vi "ATF-Sequence file decoder.vi"(8 "error in (no error)":errorcluster, 11 "file path (dialog if empty)":path) -> (0 "error out":errorcluster, 3 "Seq in":T1(array[cluster]))   [LabVIEW 2022 SP3]
uses:
  <vilib>/Utility/file.llb/Read Delimited Spreadsheet (string).vi
panel:
  in  "output cluster":T2
  out "all rows":string[][](array[string])
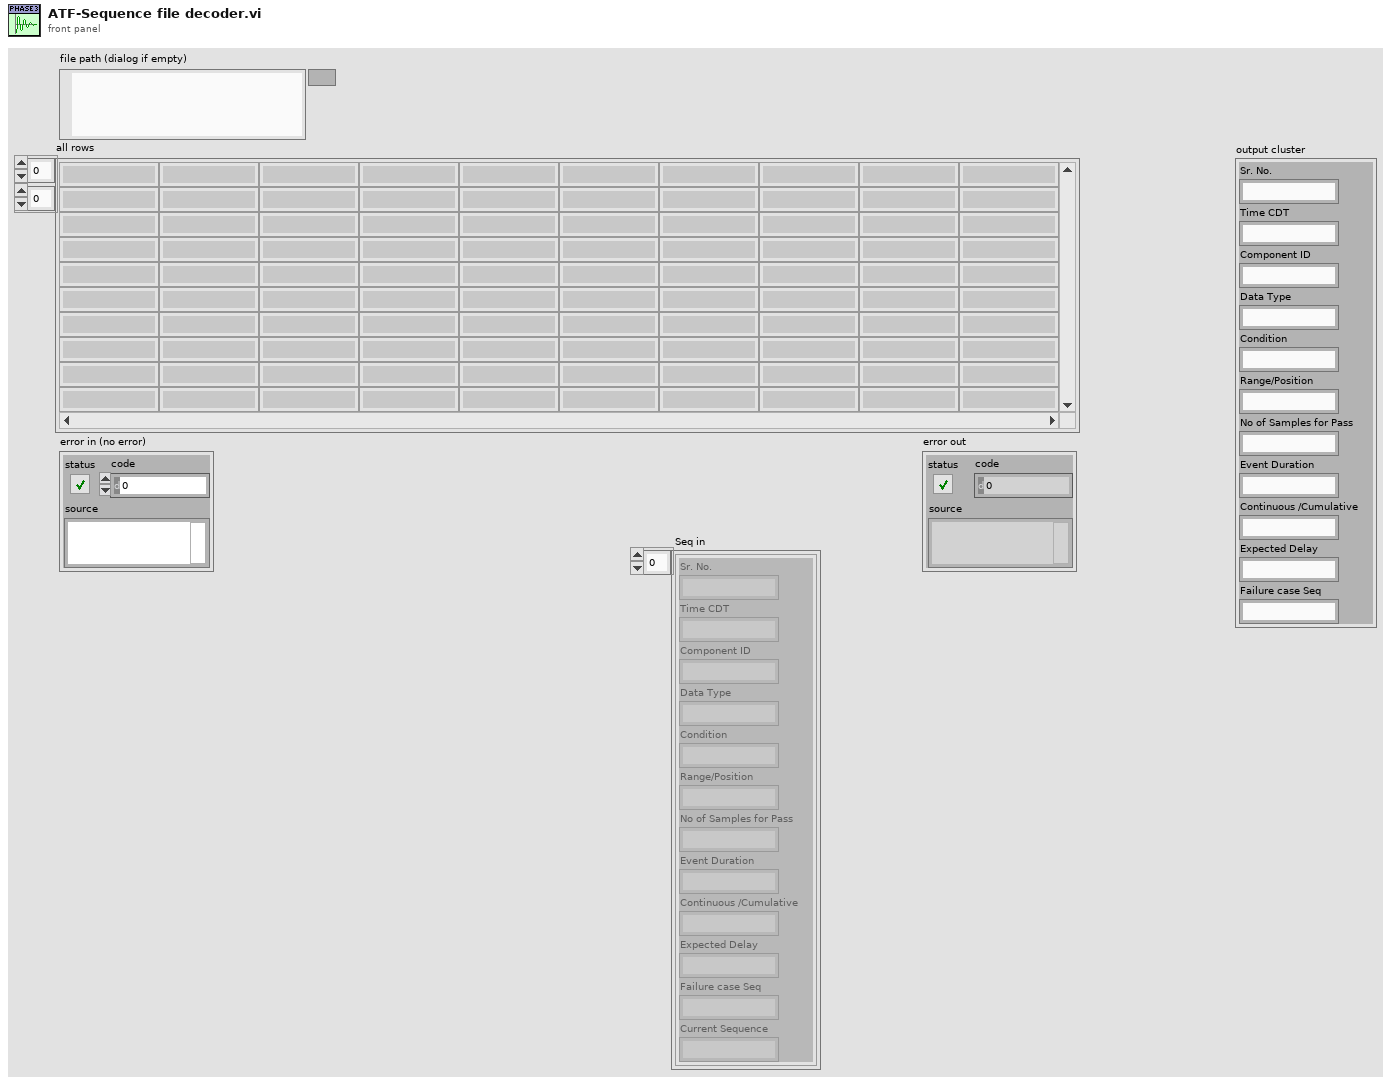
[diagram p1: front panel]
types:
  T1 = cluster{"Sr. No.":string, "Time CDT":string, "Component ID":string, "Data Type":string, "Condition":string, "Range/Position":string, "No of Samples for Pass":string, "Event Duration":string, "Continuous /Cumulative":string, "Expected Delay":string, "Failure case Seq":string, "Current Sequence":string}[]
  T2 = cluster{"Sr. No.":string, "Time CDT":string, "Component ID":string, "Data Type":string, "Condition":string, "Range/Position":string, "No of Samples for Pass":string, "Event Duration":string, "Continuous /Cumulative":string, "Expected Delay":string, "Failure case Seq":string}
  T3 = cluster{"Sr. No.":string, "Time CDT":string, "Component ID":string, "Data Type":string, "Condition":string, "Range/Position":string, "No of Samples for Pass":string, "Event Duration":string, "Continuous /Cumulative":string, "Expected Delay":string, "Failure case Seq":string, "Current Sequence":string}
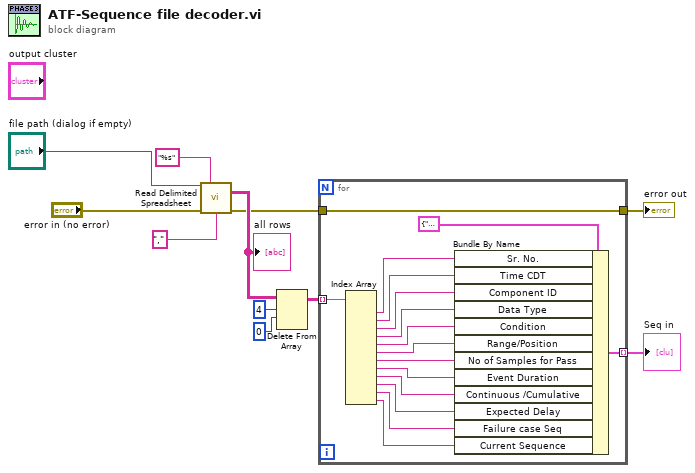
[diagram p0: block diagram]
diagram:
  n1 = call-poly <vilib>:"Read Delimited Spreadsheet.vi"("file path (dialog if empty)"="file path (dialog if empty)", "format (%s)"="%s", "error in (no error)"="error in (no error)", "delimiter (\\t)"="," ("delimiter (\\t)")) -> ("all rows"=w5:string[][], "error out"=w2:errorcluster)  [unwired: 6 in, 4 out]
  "all rows" <- w5
  n2 = Delete From Array(array=w5, length=4, index (row)=0) -> (array with subset deleted=w6:string[][])  [unwired: 1 in, 1 out]
  n3 = for {
    tunnel: w6 -> [w27] mode=indexing
    tunnel: [w20] -> w4 mode=indexing
    tunnel: w2 -> [w14]
    tunnel: [w14] -> w1
    n4 = Index Array(array=w27) -> (element #1=w26:string, element #2=w25:string, element #3=w24:string, element #4=w23:string, element #5=w22:string, element #6=w21:string, element #7=w19:string, element #8=w18:string, element #9=w17:string, element #10=w16:string, element #11=w15:string, element #12=w12:string)  [unwired: 12 in]
    n5 = Bundle By Name(cluster=T3 {"Sr. No."="", "Time CDT"="", "Component ID"="", "Data Type"="", "Condition"="", "Range/Position"="", "No of Samples for Pass"="", "Event Duration"="", "Continuous /Cumulative"="", "Expected Delay"="", "Failure case Seq"="", "Current Sequence"=""} ("output cluster"), "Sr. No."=w26, "Time CDT"=w25, "Component ID"=w24, "Data Type"=w23, "Condition"=w22, "Range/Position"=w21, "No of Samples for Pass"=w19, "Event Duration"=w18, "Continuous /Cumulative"=w17, "Expected Delay"=w16, "Failure case Seq"=w15, "Current Sequence"=w12) -> (w20:T3)
  }
  "Seq in" <- w4
  "error out" <- w1
